vi "Get Parameter Scaling.vi"(8 "error in (no error)":errorcluster, 11 "parameter ref in":T1 format="%.0x") -> (0 "error out":errorcluster, 1 "scale offset":dbl, 2 "scale multiplier":dbl, 3 "parameter ref out":T1 format="%.0x")   [LabVIEW 2020, in "AIM ARINC 429 Scripting.lvlib"]
uses:
  <vilib>/NI VeriStand/Custom Device API/Custom Device Item Ref.ctl
  AIM/Constants.vi
  <vilib>/NI VeriStand/Custom Device API/Get Item Property (Double).vi
  AIM/AIM ARINC 429 Scripting.lvlib
  <vilib>/NI VeriStand/Custom Device API/Custom Device API.lvlib
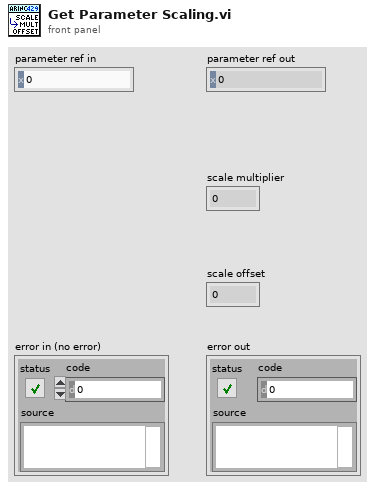
[diagram p1: front panel]
types:
  T1 = typedef "Custom Device API.lvlib/Custom Device Item Ref.ctl" = u64
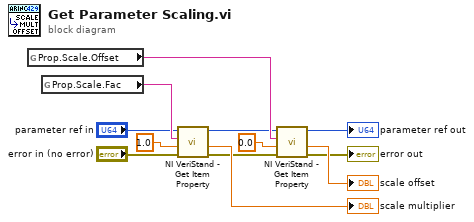
[diagram p0: block diagram]
diagram:
  n1 = global read "Constants.vi" "Prop.Scale.Offset"() -> (w8:string)
  n2 = global read "Constants.vi" "Prop.Scale.Fac"() -> (w7:string)
  n3 = call-poly <vilib>:"NI VeriStand - Get Item Property.vi"("error in (no error)"="error in (no error)", "Default Value"=1.0, "Property Name"=w7, "Item Ref in"="parameter ref in") -> ("error out"=w4:errorcluster, "Value"=→"scale multiplier":dbl, "Item Ref out"=w1:T1)  [unwired: 4 in, 1 out]
  n4 = call-poly <vilib>:"NI VeriStand - Get Item Property.vi"("error in (no error)"=w4, "Default Value"=0.0, "Property Name"=w8, "Item Ref in"=w1) -> ("error out"=→"error out":errorcluster, "Value"=→"scale offset":dbl, "Item Ref out"=→"parameter ref out":T1)  [unwired: 4 in, 1 out]
